vi "Initialize.vi"(8 "error in (no error)":errorcluster, 9 "reset device (boolean value)":bool=TRUE, 10 "Topology":string, 11 "device":refnum<k21>) -> (0 "error out":errorcluster, 3 "SLSC Switch out":refnum<class "SLSC Switch.lvclass">)   [LabVIEW 2015, in "SLSC Switch.lvclass"]
doc: "Returns a session handle used to identify the switch module in all subsequent driver calls and sets the topology of the switch module."
uses:
  SLSC Switch.lvclass
  SLSC Switch.lvclass/SLSC Switch.ctl
  <vilib>/SLSC/Initialize Session without Resources.vi
  <vilib>/SLSC/Close.vi
  <vilib>/SLSC/Close Session.vi
  <vilib>/SLSC/SLSC.lvlib
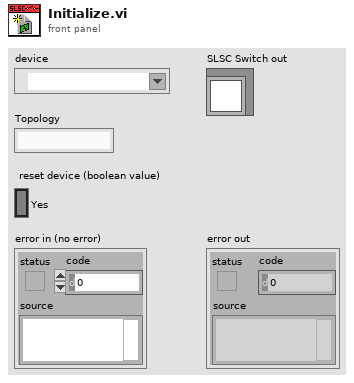
[diagram p1: front panel]
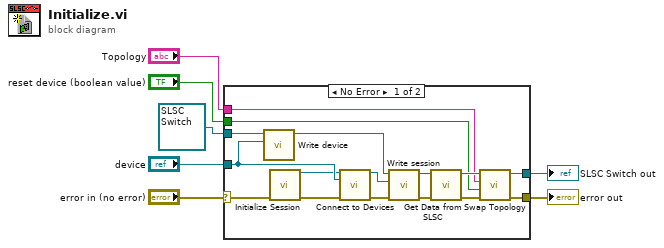
[diagram p0: block diagram]
diagram:
  n1 = case shown="No Error" "error in (no error)" {
    selector: "error in (no error)" -> [w21 w25]
    tunnel: [w9 w25] -> w6
    tunnel: refnum<class "SLSC Switch.lvclass"> refnum ("SLSC Switch in") -> [w23 w24]
    tunnel: "device" -> [w22 _]
    tunnel: "Topology" -> [w12 _]
    tunnel: "reset device (boolean value)" -> [w11 _]
    tunnel: [w8 w24] -> w1
    frame No Error {
      n2 = call "Write device.vi"("device"=w22, "SLSC Switch in"=w23) -> ("SLSC Switch out"=w20:refnum<class "SLSC Switch.lvclass">)  [unwired: 9 in]
      n3 = call-poly <vilib>:"Initialize Session.vi"("error in (no error)"=w21) -> ("session out"=w17:refnum<k21>, "error out"=w15:errorcluster)  [unwired: 13 in]
      n4 = call <vilib>:"Connect to Devices.vi"("session in"=w17, "devices"=w22, "error in (no error)"=w15) -> ("session out"=w16:refnum<k21>, "error out"=w14:errorcluster)  [unwired: 11 in]
      n5 = call "Write session.vi"("error in (no error)"=w14, "session in"=w16, "SLSC Switch in"=w20) -> ("error out"=w19:errorcluster, "SLSC Switch out"=w18:refnum<class "SLSC Switch.lvclass">)  [unwired: 7 in]
      n6 = call "Get Data from SLSC.vi"("error in (no error)"=w19, "SLSC Switch in"=w18) -> ("error out"=w10:errorcluster, "SLSC Switch out"=w13:refnum<class "SLSC Switch.lvclass">)  [unwired: 8 in]
      n7 = call "Swap Topology.vi"("error in (no error)"=w10, "reset device (boolean value)"=w11, "Topology"=w12, "SLSC Switch in"=w13) -> ("error out"=w9:errorcluster, "SLSC Switch out"=w8:refnum<class "SLSC Switch.lvclass">)  [unwired: 6 in]
    }
    frame Error {
    }
  }
  "error out" <- w6
  "SLSC Switch out" <- w1
